vi "Read Power Limits.vi"(0 "VISA resource name":refnum<visa-resource-name>, 11 "error in (no error)":errorcluster) -> (4 "VISA resource name out":refnum<visa-resource-name>, 6 "Power High Limit (V)":dbl caption="Power High Limit (W)", 8 "Power Low Limit (W)":dbl caption="Power Low Limit (V)", 15 "error out":errorcluster)   [LabVIEW 2014, in "eec 6700.lvlib"]
doc: "Reads the power limit configuration from the power source instrument.\n\nNote : Should be used in program mode only."
uses:
  <instrlib>/eec 6700/eec 6700.lvlib
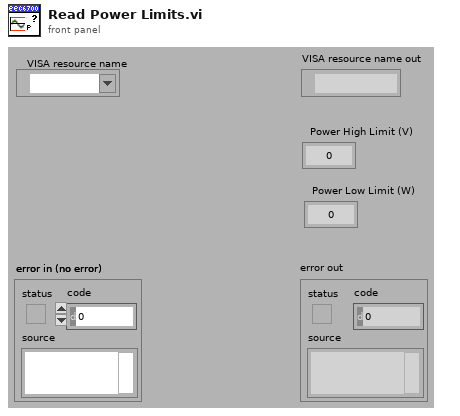
[diagram p1: front panel]
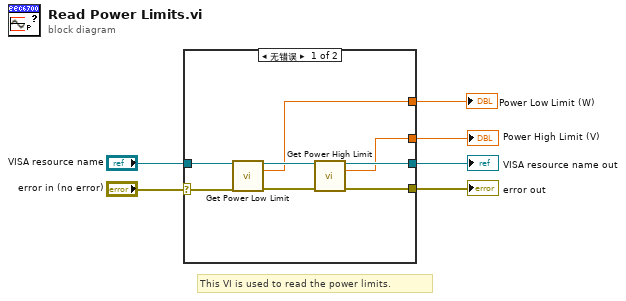
[diagram p0: block diagram]
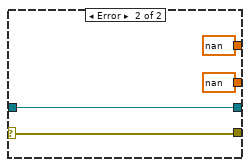
[diagram p2: hidden frame]
diagram:
  # "This VI is used to read the power limits."
  n1 = case shown="无错误" "error in (no error)" {
    selector: "error in (no error)" -> [w14 w16]
    tunnel: [w12 w16] -> w5
    tunnel: [w11 w17] -> w4
    tunnel: "VISA resource name" -> [w9 w17]
    tunnel: [w8 nan ("Voltage Low Limit")] -> w2
    tunnel: [w7 nan ("Voltage Low Limit")] -> w1
    frame No Error {
      n2 = call <instrlib>:"Get Power Low Limit.vi"("VISA resource name"=w9, "error in (no error)"=w14) -> ("VISA resource name out"=w10:refnum<visa-resource-name>, "Power Low Limit (W)"=w7:dbl, "error out"=w13:errorcluster)  [unwired: 11 in]
      n3 = call <instrlib>:"Get Power High Limit.vi"("VISA resource name"=w10, "error in (no error)"=w13) -> ("VISA resource name out"=w11:refnum<visa-resource-name>, "Power High Limit (W)"=w8:dbl, "error out"=w12:errorcluster)  [unwired: 11 in]
    }
    frame Error {
    }
  }
  "error out" <- w5
  "VISA resource name out" <- w4
  "Power High Limit (V)" <- w2
  "Power Low Limit (W)" <- w1
